vi "Get ILC Data.vi"(11 "Model in":refnum<class "Model.lvclass">) -> (2 "ILCData":T1[](array[typedef]) {"Displacement Sensor 2" format="%.4f"; "Displacement Sensor 1" format="%.4f"; "Timestamp" format="%.4f"; "Force" format="%.4f"}, 3 "Model out":refnum<class "Model.lvclass">)   [LabVIEW 2016, in "Model.lvclass"]
uses:
  Model.lvclass
  Typedefs/ActuatorData.ctl
  Model.lvclass/Model.ctl
  Typedefs/HPMT_Typedefs.lvlib
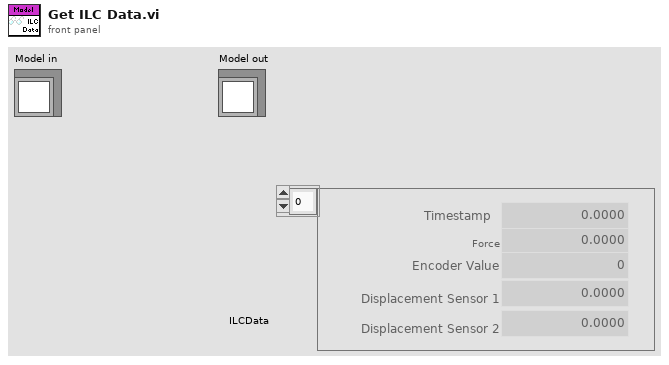
[diagram p1: front panel]
types:
  T1 = typedef "HPMT_Typedefs.lvlib/ActuatorData.ctl" = cluster{"Timestamp":dbl, "Force":dbl, "Encoder Value":i32, "Displacement Sensor 1":dbl, "Displacement Sensor 2":dbl}
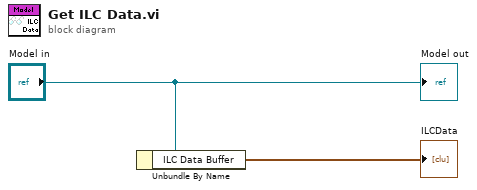
[diagram p0: block diagram]
diagram:
  n1 = Unbundle By Name("Model in") -> ("ILC Data Buffer"=→"ILCData":T1[])
  "Model out" <- "Model in"
